vi "test_Read SGL Register Value.vi"(8 "error in (no error)":errorcluster, 11 "TestCase in":refnum<class "FPGA Register IO Tests.lvclass">) -> (0 "error out":errorcluster, 3 "TestCase out":refnum<class "FPGA Register IO Tests.lvclass">)   [LabVIEW 2021, in "FPGA Register IO Tests.lvclass"]
uses:
  FPGA Register IO Tests.lvclass
  FPGA Register IO Tests.lvclass/FPGA Register IO Tests.ctl
  APIs/FPGA Register IO/Read Methods/Read Data Register/Instances/Read SGL.vi
  APIs/FPGA Register IO/Utilities/Find Register Offset.vi
  APIs/FPGA Register IO/SubVIs/Check Register Data Store.vi
  APIs/FPGA Register IO/Error Handling/Error 6001.vi
  APIs/FPGA Register IO/Error Handling/Error 6000.vi
  APIs/FPGA Register IO/Error Handling/Error 6002.vi
  APIs/FPGA Register IO/Error Handling/Error 6003.vi
  <vilib>/FPGAPlugInAG/Dynamic/niLvFpga_Close_Dynamic.vi
  <vilib>/rvi/interface/nirviCloseFPGA/nirviCloseFPGA.xnode
  <vilib>/addons/_JKI Toolkits/VI Tester/TestCase.llb/TestCase.lvclass
  APIs/FPGA Register IO/FPGA Register IO.lvlib
  C:/Program Files/National Instruments/LabVIEW 2021/vi.lib/addons/_JKI Toolkits/VI Tester/TestCase.llb/TestCase.lvclass
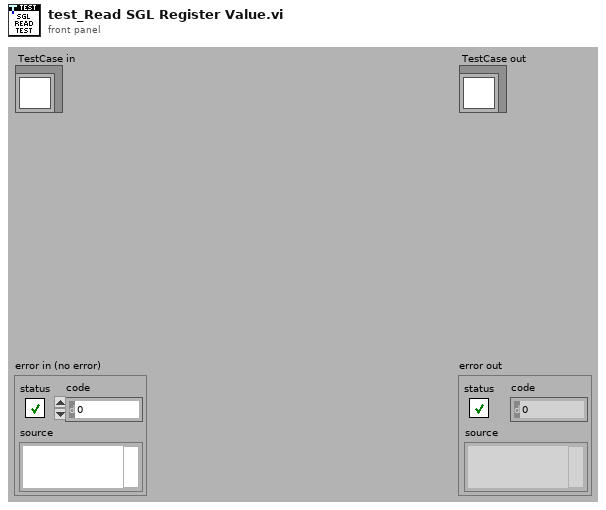
[diagram p1: front panel]
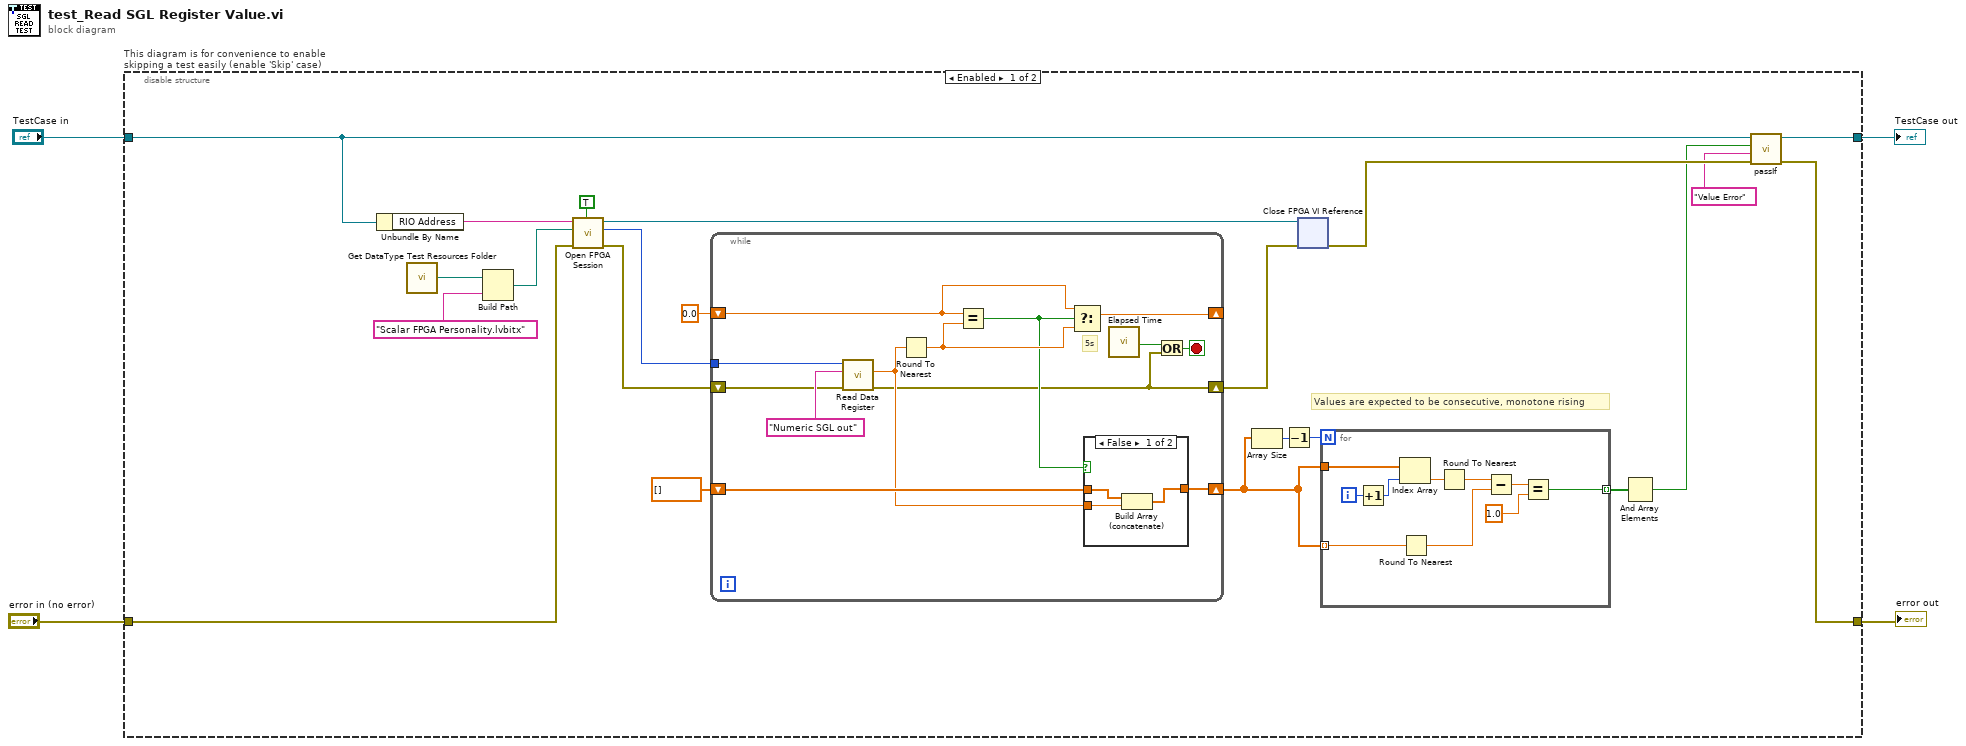
[diagram p0: block diagram]
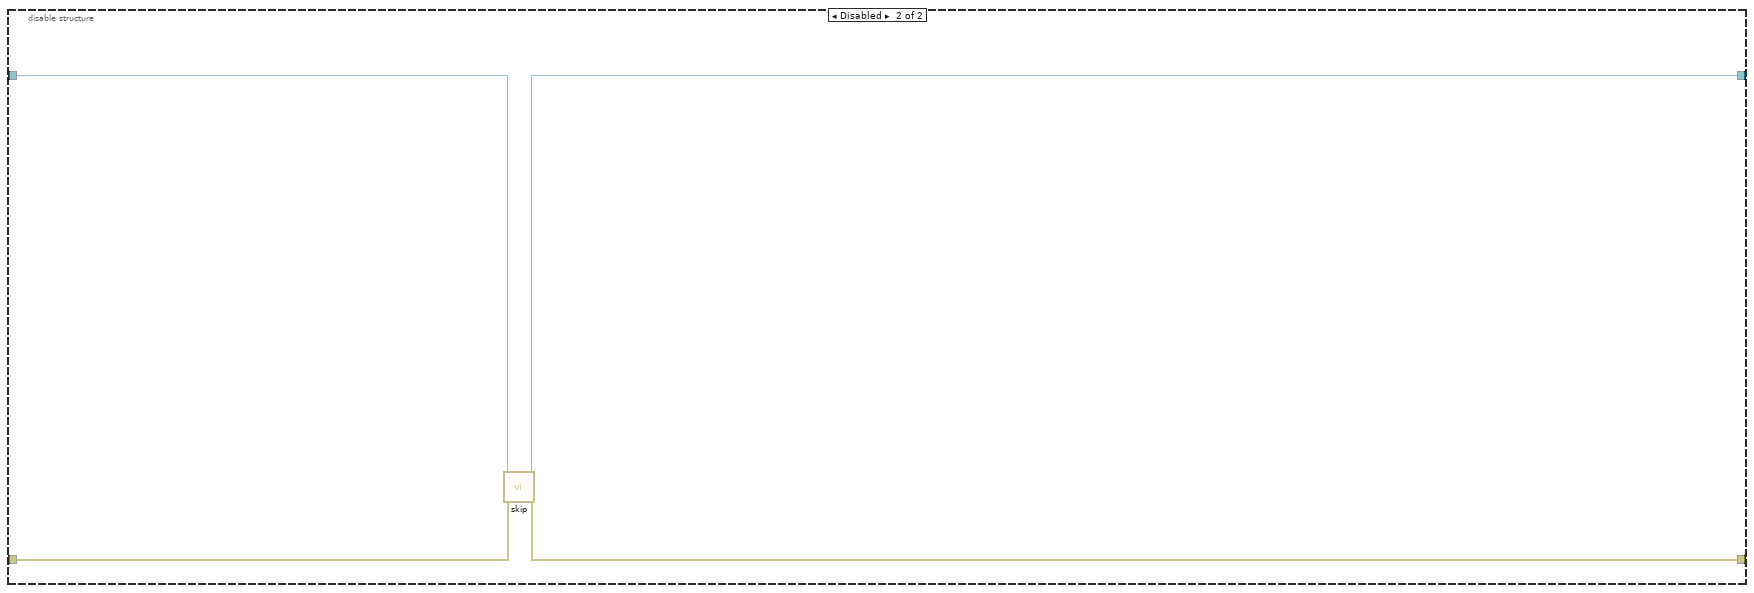
[diagram p3: hidden frame]
diagram:
  n1 = disable-structure "This diagram is for convenience to enable skipping a test easily (enable 'Skip' case)" shown="Enabled" {
    disable-tunnel: "TestCase in" -> [w12 w57]
    disable-tunnel: [w6 w55] -> w1
    disable-tunnel: [w5 w56] -> w3
    disable-tunnel: "error in (no error)" -> [w13 w54]
    frame Enabled {
      # "Values are expected to be consecutive, monotone rising"
      n2 = Unbundle By Name(w12) -> ("RIO Address"=w15:string)
      n3 = call "Get DataType Test Resources Folder.vi"() -> ("path"=w10:path)
      n4 = Build Path(base path=w10, name or relative path="Scalar FPGA Personality.lvbitx") -> (appended path=w14:path)
      n5 = call "Open FPGA Session.vi"("run when loaded (T)"=TRUE ("Run When Loaded (T)"), "error in"=w13, "bitfile path"=w14, "device address"=w15) -> ("error out"=w21:errorcluster, "session out"=w20:u32, "bitfile reference out"=w19:refnum<k20>)  [unwired: 5 in]
      n6 = while {
        tunnel: w20 -> [w33]
        shift-right: [w27] -> w18
        shift-left: w21 -> [w31]
        shift-right: [w37] -> _
        shift-left: sgl 0.0 ("DBL Value") -> [w39]
        shift-right: [w35] -> w22
        shift-left: sgl[] [] -> [w34]
        stop <- w29 stop-if-true
        # "5s"
        n7 = call-poly "Read Data Register.vi"("error in"=w31, "register name"="Numeric SGL out" ("registerName"), "session in"=w33) -> ("error out"=w27:errorcluster, "value out"=w30:sgl)  [unwired: 6 in, 1 out]
        n8 = Round To Nearest(number=w30) -> (nearest integer value=w38:sgl)
        n9 = Equal?(x=w39, y=w38) -> (x = y?=w36:bool)
        n10 = Select(t=w39, s=w36, f=w38) -> (s? t:f=w37:sgl)
        n11 = case shown="False" w36 {
          tunnel: w30 -> [w42 _]
          tunnel: [w41 w43] -> w35
          tunnel: w34 -> [w40 w43]
          frame False {
            n12 = Build Array (concatenate)(w40, w42) -> (w41:sgl[])
          }
          frame True {
          }
        }
        n13 = call "Elapsed Time"() -> ("Time has Elapsed"=w28:bool)  [unwired: 12 in, 7 out]
        n14 = Or(x=w28, y=w27) -> (x .or. y?=w29:bool)
      }
      n15 = Array Size(array=w22) -> (size(s)=w23:i32)
      n16 = Decrement(x=w23) -> (x-1=w24:i32)
      n17 = xnode "Close FPGA VI Reference"("FPGA VI Reference In"=w19, "error in"=w18) -> ("error out"=w11:errorcluster)
      n18 = for {
        N: w24 -> [_]
        tunnel: w22 -> [w48] mode=indexing
        tunnel: w22 -> [w53]
        tunnel: [w44] -> w25 mode=indexing
        i -> [w52]
        n19 = Increment(x=w52) -> (x+1=w51:i32)
        n20 = Index Array(array=w53, index=w51) -> (element=w50:sgl)
        n21 = Round To Nearest(number=w48) -> (nearest integer value=w47:sgl)
        n22 = Round To Nearest(number=w50) -> (nearest integer value=w49:sgl)
        n23 = Subtract(x=w49, y=w47) -> (x-y=w46:sgl)
        n24 = Equal?(x=w46, y=sgl 1.0) -> (x = y?=w44:bool)
      }
      n25 = And Array Elements(Boolean array=w25) -> (logical AND=w9:bool)
      n26 = call-dynamic "passIf.vi"("error in (no error)"=w11, "message (\"\")"="Value Error" ("message (\"\")"), "pass"=w9, "TestCase in"=w12) -> ("error out"=w5:errorcluster, "TestCase out"=w6:refnum<class "FPGA Register IO Tests.lvclass">)  [unwired: 6 in]
    }
    frame Disabled {
      # "skip test result while test is under development"
      n27 = call <vilib>:"skip.vi"("error in (no error)"=w54, "TestCase in"=w57) -> ("error out"=w56:errorcluster, "TestCase out"=w55:refnum<class "FPGA Register IO Tests.lvclass">)  [unwired: 8 in]
    }
  }
  "error out" <- w3
  "TestCase out" <- w1
